vi "Pruebas.vi"() -> ()   [LabVIEW 2020]
uses:
  f4c0b859-3fa6-4875-91a9-a1890523c36e.vi
panel:
  out "bool response":bool[](array[boolean])
  out "error out":errorcluster
  in  "error in (no error)":errorcluster
  in  "stop":bool
  in  "Boolean":bool
  in  "String 2":string
  out "String":string
  in  "VISA resource name":refnum<visa-resource-name>
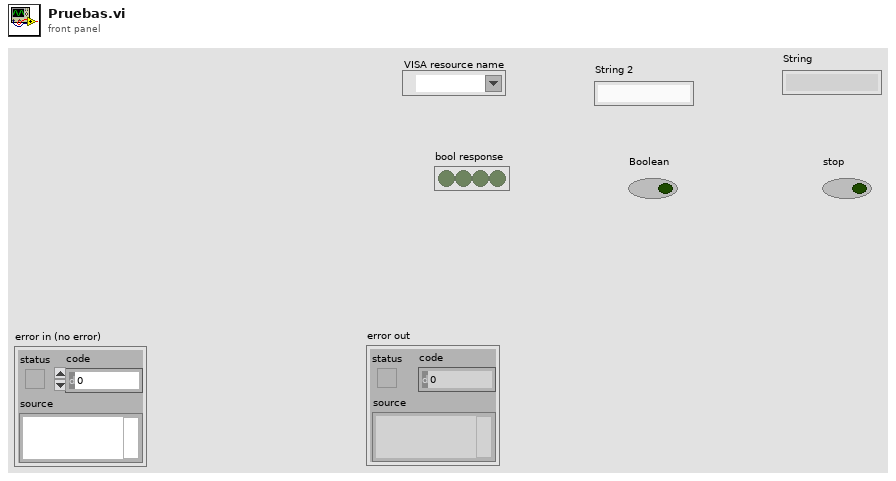
[diagram p1: front panel]
types:
  T1 = enum16{"Write", "Read", "Config", "Reset", "Close"}
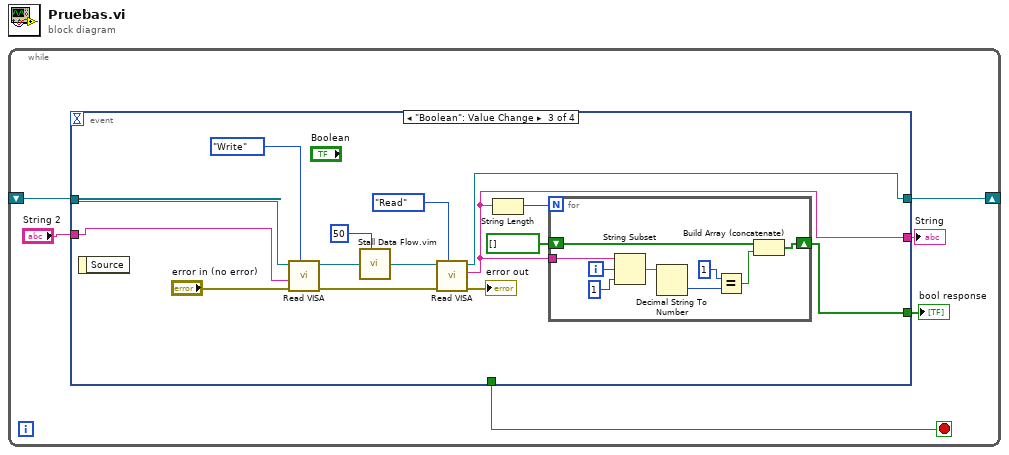
[diagram p0: block diagram]
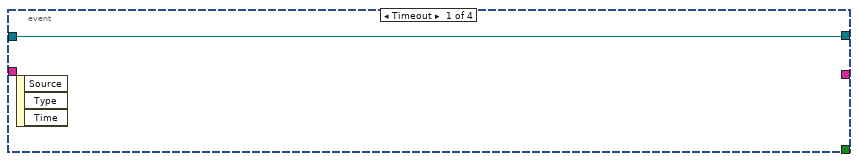
[diagram p2: hidden frame]
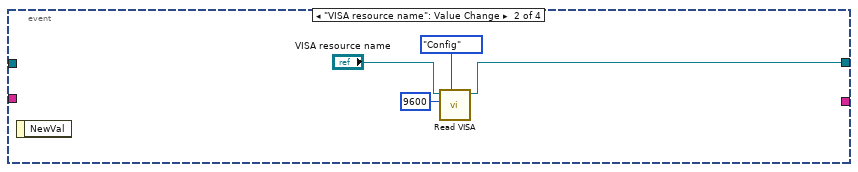
[diagram p3: hidden frame]
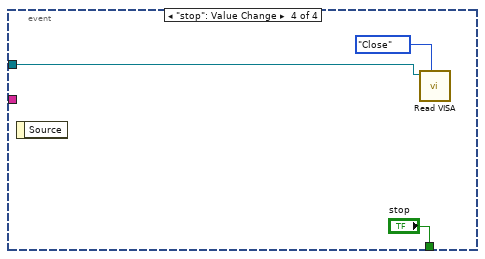
[diagram p4: hidden frame]
diagram:
  n1 = while {
    shift-right: [w6] -> _
    shift-left: _ -> [w5]
    stop <- w2 stop-if-true
    n2 = event shown="[2] \"Boolean\": Value Change" {
      selector: _ -> [_ _ _ _]
      dyn-events: _ -> [_ _ _ _]
      timeout: _ -> [_ _ _ _]
      tunnel: [w7 w10 w15 _] -> w6
      tunnel: w5 -> [w7 _ w16 w37]
      tunnel: "String 2" -> [_ _ w17 _]
      tunnel: [_ _ w13 _] -> w3
      tunnel: [_ _ _ "stop"] -> w2
      tunnel: [_ _ w14 _] -> w1
      event Timeout {
        n3 = event-data() -> ()  [unwired: 1 in, 3 out]
      }
      event "VISA resource name": Value Change {
        n4 = event-data() -> ()  [unwired: 1 in, 1 out]
        n5 = call "Read VISA.vi"("Opciones"=T1."Config", "baud rate (9600)"=u32 9600, "VISA com port"="VISA resource name") -> ("VISA com port 2"=w10:refnum<visa-resource-name>)  [unwired: 6 in, 2 out]
      }
      event "Boolean": Value Change {
        n6 = event-data() -> ()  [unwired: 1 in, 1 out]
        n7 = call "Read VISA.vi"("Opciones"=T1."Write", "error in (no error)"="error in (no error)", "Write"=w17, "VISA com port"=w16) -> ("error out"=w22:errorcluster, "VISA com port 2"=w25:refnum<visa-resource-name>)  [unwired: 5 in, 1 out]
        n8 = call "Stall Data Flow.vim"("value in"=w25, "milliseconds to wait"=u32 50) -> ("value out"=w24:refnum<visa-resource-name>)  [unwired: 1 out]
        n9 = call "Read VISA.vi"("Opciones"=T1."Read", "error in (no error)"=w22, "VISA com port"=w24) -> ("error out"=→"error out":errorcluster, "Read"=w13:string, "VISA com port 2"=w15:refnum<visa-resource-name>)  [unwired: 6 in]
        n10 = String Length(string=w13) -> (length=w18:i32)
        n11 = for {
          N: w18 -> [_]
          tunnel: w13 -> [w35]
          shift-right: [w28] -> w14
          shift-left: bool[] [] -> [w27]
          i -> [w34]
          n12 = String Subset(string=w35, offset (0)=w34, length (rest)=1 ("length (rest)")) -> (substring=w32:string)
          n13 = Decimal String To Number(string=w32) -> (number=w31:i32)  [unwired: 2 in, 1 out]
          n14 = Equal?(x=1, y=w31) -> (x = y?=w29:bool)
          n15 = Build Array (concatenate)(w27, w29) -> (w28:bool[])
        }
      }
      event "stop": Value Change {
        n16 = event-data() -> ()  [unwired: 1 in, 1 out]
        n17 = call "Read VISA.vi"("Opciones"=T1."Close", "VISA com port"=w37) -> ()  [unwired: 7 in, 3 out]
      }
    }
    "String" <- w3
    "bool response" <- w1
  }
